vi "CML Main.vi"() -> ()   [LabVIEW 2017]
doc: "_____\nBased on Delacor QMH Project Template 4.1.0.56."
uses:
  Libraries/CML UI/CML UI.lvlib
panel:
  out "Command Line Arguments":string[](array[string])
  out "Module Running?":bool
  out "Status":string
  out "error out":errorcluster
  in  "Stop Module":bool
  in  "Start Module":bool
  # "See the Build_Final_EXE bookmarks on the diagram for instructions on using this VI as a launcher for an EXE."
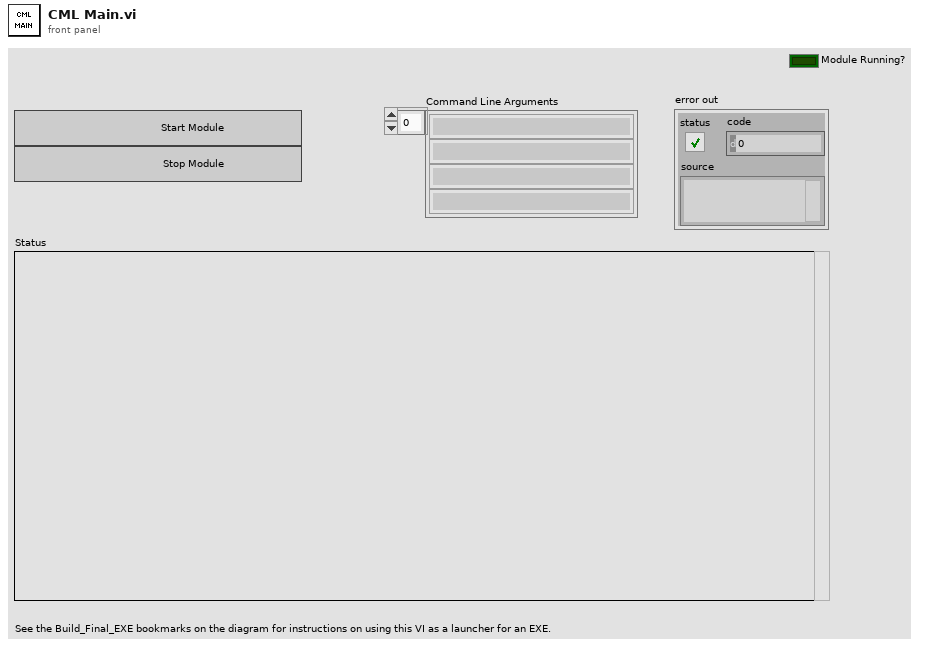
[diagram p1: front panel]
types:
  T1 = typedef "CML UI.lvlib/Broadcast Events--cluster.ctl" = cluster{"Module Did Init":refnum<user-event>, "Status Updated":refnum<user-event>, "Error Reported":refnum<user-event>, "Module Did Stop":refnum<user-event>, "Update Module Execution Status":refnum<user-event>}
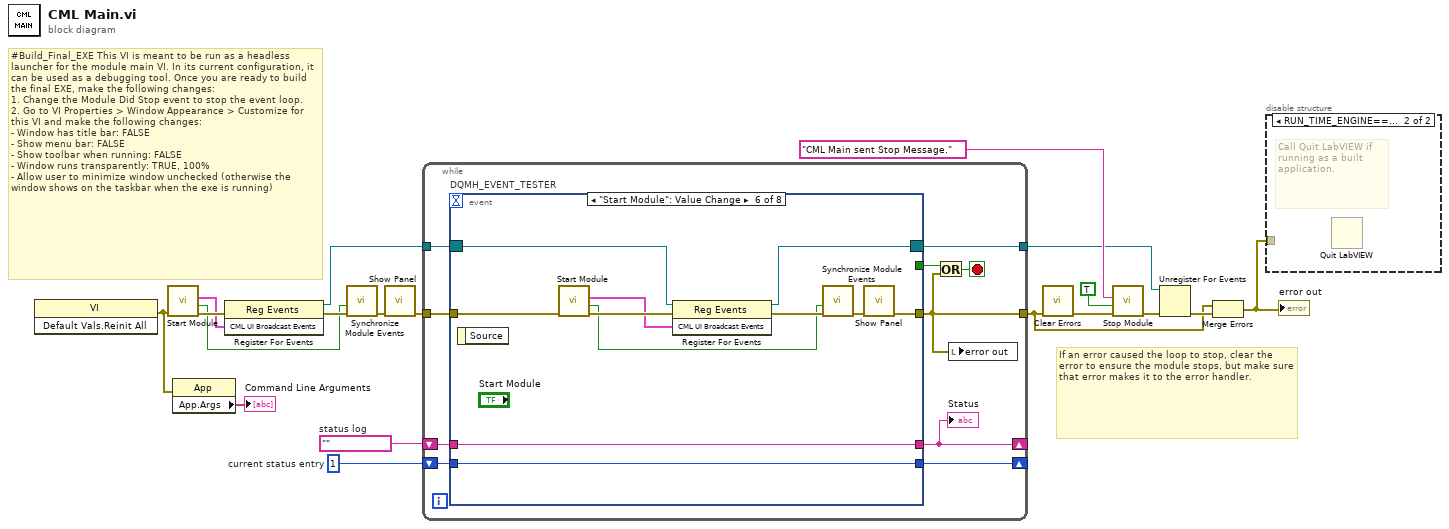
[diagram p0: block diagram]
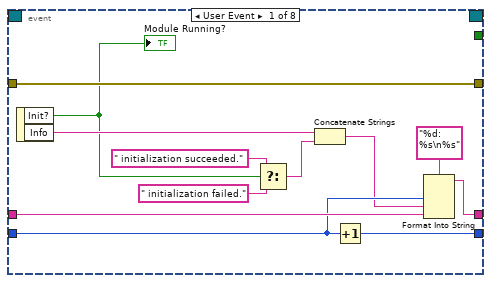
[diagram p2: hidden frame]
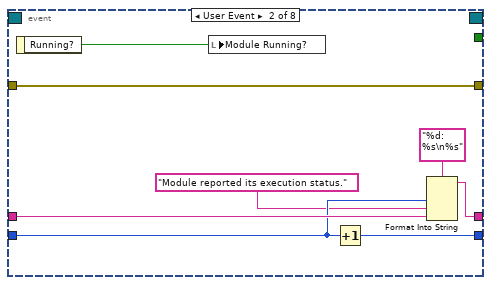
[diagram p3: hidden frame]
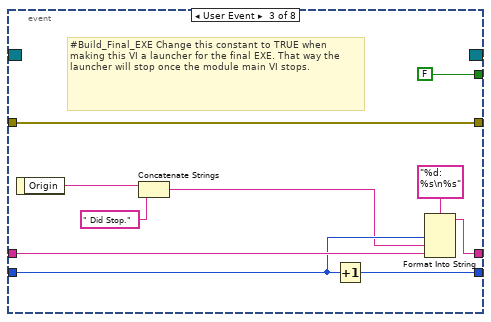
[diagram p4: hidden frame]
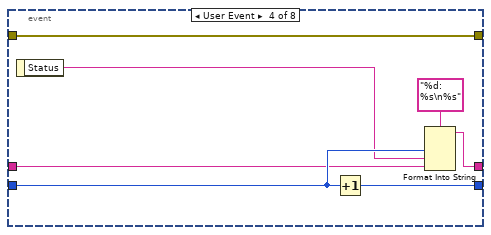
[diagram p5: hidden frame]
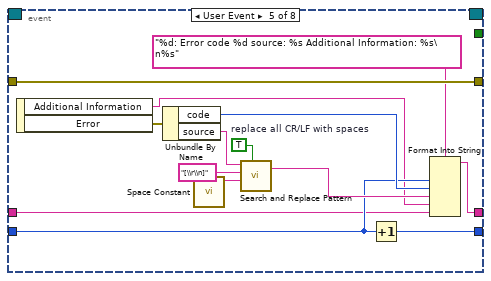
[diagram p6: hidden frame]
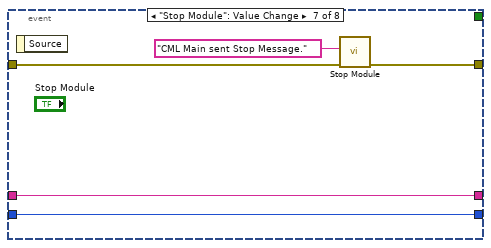
[diagram p7: hidden frame]
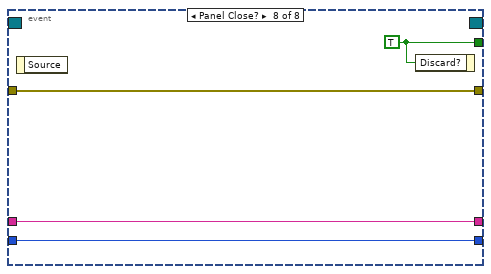
[diagram p8: hidden frame]
diagram:
  w15 = 1  # current status entry
  w16 = ""  # status log
  # "#Build_Final_EXE This VI is meant to be run as a headless launcher for the module main VI. In its current configuration, it can be used as a debugging tool. Once you are ready to build the final EXE, make the following changes:\n1. Change the Module Did Stop event to stop the event loop.\n2. Go to VI Properties > Window Appearance > Customize for this VI and make the following changes:\n- Window has title bar: FALSE\n- Show menu bar: FALSE\n- Show toolbar when running: FALSE\n- Window runs transparently: TRUE, 100%\n- Allow user to minimize window unchecked (otherwise the window shows on the taskbar when the exe is running)"
  # "If an error caused the loop to stop, clear the error to ensure the module stops, but make sure that error makes it to the error handler."
  n1 = invoke on="Invoke Node" class="VI" method="Default Vals.Reinit All"() -> (error out=w1:errorcluster)  [unwired: 3 in, 2 out]
  n2 = call "Start Module.vi"("error in (no error)"=w1) -> ("error out"=w10:errorcluster, "Wait for Event Sync?"=w9:bool, "CML UI Broadcast Events"=w8:T1)  [unwired: 7 in, 1 out]
  n3 = property on="Property Node" class="App"(error in=w1) -> ("App.Args"=→"Command Line Arguments":string[])  [unwired: 1 in, 2 out]
  n4 = register-events(error in=w10, w8) -> (reference out=w7:refnum<event-registration>, error out=w11:errorcluster)  [unwired: 1 in]
  n5 = call "Synchronize Module Events.vi"("error in (no error)"=w11, "Wait for Event Sync?"=w9) -> ("error out"=w5:errorcluster)  [unwired: 9 in]
  n6 = call "Show Panel.vi"("error in (no error)"=w5) -> ("error out"=w4:errorcluster)  [unwired: 10 in]
  n7 = while {
    tunnel: w7 -> [w29]
    tunnel: [w20] -> w3
    shift-right: [w21] -> _
    shift-left: w16 -> [w26]
    shift-right: [w25] -> _
    shift-left: w15 -> [w27]
    tunnel: w4 -> [w23]
    tunnel: [w22] -> w14
    stop <- w24 stop-if-true
    n8 = event "DQMH_EVENT_TESTER" shown="[5] \"Start Module\": Value Change" {
      selector: w29 -> [_ _ _ _ _ w85 _ _]
      dyn-events: [_ _ _ _ _ w84 _ _] -> w22
      timeout: _ -> [_ _ _ _ _ _ _ _]
      tunnel: [_ _ FALSE ("Discard?") _ _ _ _ w100] -> w28
      tunnel: [w41 w43 w51 w60 w80 w81 w94 w97] -> w20
      tunnel: w27 -> [w38 w47 w57 w63 w70 w88 w95 w98]
      tunnel: w26 -> [w39 w48 w58 w62 w68 w89 w96 w99]
      tunnel: [w36 w45 w55 w64 w71 w89 w96 w99] -> w21
      tunnel: [w37 w46 w56 w66 w69 w88 w95 w98] -> w25
      tunnel: w23 -> [w41 w43 w51 w60 w80 w83 w92 w97]
      event User Event {
        n9 = event-data() -> ("Init?"=w33:bool, "Info"=w35:string)  [unwired: 1 in]
        "Module Running?" <- w33
        n10 = Select(t=" initialization succeeded.", s=w33, f=" initialization failed.") -> (s? t:f=w30:string)
        n11 = Concatenate Strings(w35, w30) -> (w34:string)
        n12 = Increment(x=w38) -> (x+1=w37:i32)
        n13 = Format Into String(format string="%d: %s\n%s", w38, w34, w39) -> (resulting string=w36:string)  [unwired: 2 in, 1 out]
      }
      event User Event {
        n14 = event-data() -> ("Running?"=w42:bool)  [unwired: 1 in]
        n15 = local write "Module Running?"(w42) -> ()
        n16 = Increment(x=w47) -> (x+1=w46:i32)
        n17 = Format Into String(format string="%d: %s\n%s", w47, "Module reported its execution status.", w48) -> (resulting string=w45:string)  [unwired: 2 in, 1 out]
      }
      event User Event {
        # "#Build_Final_EXE Change this constant to TRUE when making this VI a launcher for the final EXE. That way the launcher will stop once the module main VI stops."
        n18 = event-data() -> ("Origin"=w54:string)  [unwired: 1 in]
        n19 = Concatenate Strings(w54, " Did Stop.") -> (w53:string)
        n20 = Increment(x=w57) -> (x+1=w56:i32)
        n21 = Format Into String(format string="%d: %s\n%s", w57, w53, w58) -> (resulting string=w55:string)  [unwired: 2 in, 1 out]
      }
      event User Event {
        n22 = event-data() -> ("Status"=w61:string)  [unwired: 1 in]
        n23 = Increment(x=w63) -> (x+1=w66:i32)
        n24 = Format Into String(format string="%d: %s\n%s", w63, w61, w62) -> (resulting string=w64:string)  [unwired: 2 in, 1 out]
      }
      event User Event {
        w76 = TRUE  # replace all CR/LF with spaces
        n25 = event-data() -> ("Additional Information"=w67:string, "Error"=w72:errorcluster)  [unwired: 1 in]
        n26 = Unbundle By Name(w72) -> ("code"=w73:i32, "source"=w74:string)
        n27 = call <vilib>:"Space Constant.vi"() -> ("String"=w77:string)
        n28 = call <vilib>:"Search and Replace Pattern.vi"("string"=w74, "regular expression (\"\")"="[\\r\\n]" ("regular expression (\"\")"), "replace string (\"\")"=w77, "replace all? (F)"=w76) -> ("result string"=w75:string)  [unwired: 1 in, 1 out]
        n29 = Increment(x=w70) -> (x+1=w69:i32)
        n30 = Format Into String(format string="%d: Error code %d source: %s Additional Information: %s\n%s", w70, w73, w75, w67, w68) -> (resulting string=w71:string)  [unwired: 2 in, 1 out]
      }
      event "Start Module": Value Change {
        n31 = event-data() -> ()  [unwired: 1 in, 1 out]
        n32 = call "Start Module.vi"("error in (no error)"=w83) -> ("error out"=w90:errorcluster, "Wait for Event Sync?"=w87:bool, "CML UI Broadcast Events"=w86:T1)  [unwired: 7 in, 1 out]
        n33 = register-events(reference=w85, error in=w90, w86) -> (reference out=w84:refnum<event-registration>, error out=w91:errorcluster)
        n34 = call "Synchronize Module Events.vi"("error in (no error)"=w91, "Wait for Event Sync?"=w87) -> ("error out"=w82:errorcluster)  [unwired: 9 in]
        n35 = call "Show Panel.vi"("error in (no error)"=w82) -> ("error out"=w81:errorcluster)  [unwired: 10 in]
      }
      event "Stop Module": Value Change {
        n36 = event-data() -> ()  [unwired: 1 in, 1 out]
        n37 = call "Stop Module.vi"("error in (no error)"=w92, "Origin"="CML Main sent Stop Message.") -> ("error out"=w94:errorcluster)  [unwired: 9 in]
      }
      event Panel Close? {
        w100 = TRUE ("Discard?")
        n38 = event-data() -> ()  [unwired: 1 in, 1 out]
        n39 = event-data ("Event Filter Node")("Discard?"=w100) -> ()  [unwired: 1 in, 1 out]
      }
    }
    "Status" <- w21
    n40 = Or(x=w28, y=w20) -> (x .or. y?=w24:bool)
    n41 = local write "error out"(w20) -> ()
  }
  n42 = call <vilib>:"Clear Errors.vi"("error in (no error)"=w3) -> ("error out"=w12:errorcluster)  [unwired: 5 in, 1 out]
  n43 = call "Stop Module.vi"("error in (no error)"=w12, "Wait for Module to Stop? (F)"=TRUE ("Wait for Module to stop?"), "Origin"="CML Main sent Stop Message.") -> ("error out"=w18:errorcluster)  [unwired: 8 in]
  n44 = Unregister For Events(event registration refnum=w14, error in=w18) -> (error out=w19:errorcluster)
  n45 = Merge Errors(w3, w19) -> (w6:errorcluster)
  "error out" <- w6
  n46 = disable-structure "Conditional Disable Structure" shown="RUN_TIME_ENGINE==True" {
    disable-tunnel: w6 -> [_ _]
    frame condition #0 (active) {
    }
    frame condition #1 {
      # "Call Quit LabVIEW if running as a built application."
      n47 = Quit LabVIEW() -> ()  [unwired: 1 in]
    }
  }
